vi "niTuner Initiate Scan.vi"(8 "error in":errorcluster, 11 "taskID in":i32 format="%.0x") -> (0 "error out":errorcluster, 3 "taskID out":i32 format="%.0x")   [LabVIEW 2011]
doc: "This VI readies the PXI-5600 downconverter to begin settling to the first frequency entry in the scan list. If a ready trigger is configured, the ready trigger is generated after the PXI-5600 downconverter has settled."
uses:
  nipxi5600u.dll
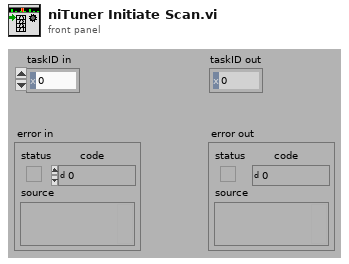
[diagram p1: front panel]
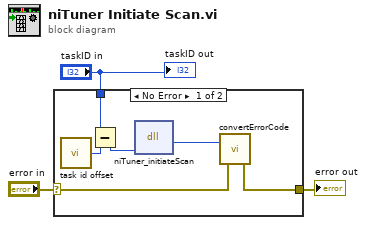
[diagram p0: block diagram]
diagram:
  n1 = case shown="No Error" "error in" {
    selector: "error in" -> [w8 w10]
    tunnel: [w7 w10] -> w2
    tunnel: "taskID in" -> [w4 _]
    frame No Error {
      n2 = call <instrlib>:"task id offset.vi"() -> ("taskID offset"=w5:i32)
      n3 = Subtract(x=w4, y=w5) -> (x-y=w6:i32)
      n4 = dll-call lib="nipxi5600u.dll" fn="niTuner_initiateScan"("taskID"=w6) -> (w9:i32)  [unwired: 4 in, 2 out]
      n5 = call <instrlib>:"convertErrorCode.vi"("error in"=w8, "error code"=w9) -> ("error out"=w7:errorcluster)
    }
    frame Error {
    }
  }
  "error out" <- w2
  "taskID out" <- "taskID in"
